vi "Read CSV File.vi"(7 "delimiter (,)":string=",", 8 "error in (no error)":errorcluster, 11 "file path in":path) -> (0 "error out":errorcluster, 2 "2-D array":string[][](array[string]), 3 "file path out":path)   [LabVIEW 2013, in "Robust CSV.lvlib"]
doc: "Reads a CSV (Character Separated Values) spreadsheet file to a 2D array of strings.\nThe CSV spreadsheet is assumed to be ANSI encoded and formatted in accordance with RFC-4180 (see http://tools.ietf.org/html/rfc4180). \nAll EOLs (CR, LF or CR+LF) will be converted to LF and all escaped double quotes will be un-escaped in the output array.\n\nRev 0.0 2014-02-20 Ryan Porter\nFirst Draft"
uses:
  Robust CSV.lvlib
panel:
  # "Read CSV File.vi\n\nReads a CSV (Character Separated Values) spreadsheet file to a 2D array of strings.\nThe CSV spreadsheet is assumed to be ANSI encoded and formatted in accordance with RFC-4180 (see http://tools.ietf.org/html/rfc4180). \nAll EOLs (CR, LF or CR+LF) will be converted to LF and all escaped double quotes will be un-escaped in the output array."
  # "License: BSD (2-Clause) - http://opensource.org/licenses/BSD-2-Clause \n\nCopyright (c) 2014, Ryan Porter\nAll rights reserved."
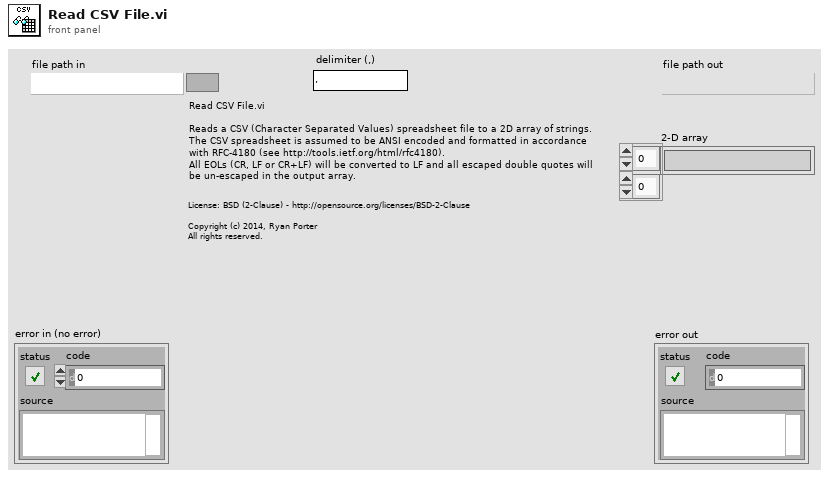
[diagram p1: front panel]
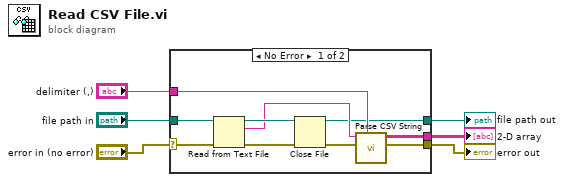
[diagram p0: block diagram]
diagram:
  n1 = case shown="No Error" "error in (no error)" {
    selector: "error in (no error)" -> [w13 w17]
    tunnel: "file path in" -> [w14 w18]
    tunnel: [w7 _] -> w2
    tunnel: "delimiter (,)" -> [w11 _]
    tunnel: [w10 w18] -> w3
    tunnel: [w8 w17] -> w1
    frame No Error {
      n2 = Read from Text File(file (use dialog)=w14, error in=w13) -> (refnum out=w16:refnum<file>, text=w12:string, error out=w15:errorcluster)  [unwired: 2 in, 1 out]
      n3 = Close File(refnum=w16, error in=w15) -> (path=w10:path, error out=w9:errorcluster)
      n4 = call "Parse CSV String.vi"("delimiter (,)"=w11, "error in"=w9, "CSV string"=w12) -> ("error out"=w8:errorcluster, "2-D array"=w7:string[][])  [unwired: 7 in]
    }
    frame Error {
    }
  }
  "2-D array" <- w2
  "error out" <- w1
  "file path out" <- w3
